vi "windows media player run.vi"() -> ()   [LabVIEW 2020]
panel:
  in  "File Path":path
  in  "WindowsMediaPlayer":refnum<k7>(container)
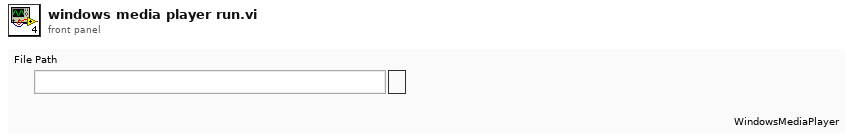
[diagram p1: front panel]
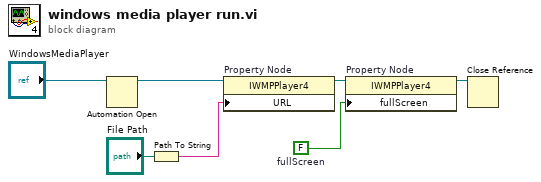
[diagram p0: block diagram]
diagram:
  w3 = FALSE  # fullScreen
  n1 = Automation Open(Automation Refnum="WindowsMediaPlayer") -> (Automation Refnum=w6:refnum<k7>)  [unwired: 3 in, 1 out]
  n2 = Path To String(path="File Path") -> (string=w5:string)
  n3 = property on="Property Node" class="IWMPPlayer4"(reference=w6, "URL"=w5) -> (reference out=w2:refnum<k7>)  [unwired: 1 in, 1 out]
  n4 = property on="Property Node" class="IWMPPlayer4"(reference=w2, "fullScreen"=w3) -> (reference out=w1:refnum<k7>)  [unwired: 1 in, 1 out]
  n5 = Close Reference(reference=w1) -> ()  [unwired: 1 in, 1 out]
